vi "Configure Surge-Drop Duration.vi"(0 "VISA resource name":refnum<visa-resource-name>, 5 "Surge Drop Duration (0 ms)":dbl min=0.0 max=99.0, 11 "error in (no error)":errorcluster) -> (4 "VISA resource name out":refnum<visa-resource-name>, 15 "error out":errorcluster)   [LabVIEW 2020, in "eec 6700.lvlib"]
doc: "Sets <B>surge drop duration</B> of the power source instrument.\n\n<B>Range</B> : \nIf Surge Drop Continuous = ON : 0 ~ 20ms\nIf Surge Drop Continuous = OFF : 0 ~ 99ms\n\nThe Surge Drop-Time parameter setting configures the overall time duration of the surge or drop voltage. For example if the Surge Drop-Site is 50 milliseconds; the output voltage is 120 volts; the surge voltage is 150 volts; and the Surge Drop-Time is 20 milliseconds when the sine wave reaches the 50 millisecond point (180º) the voltage will surge to 150 volts. This surge will hold for 20 milliseconds before the voltage output returns to 120 volts"
uses:
  <instrlib>/eec 6700/eec 6700.lvlib
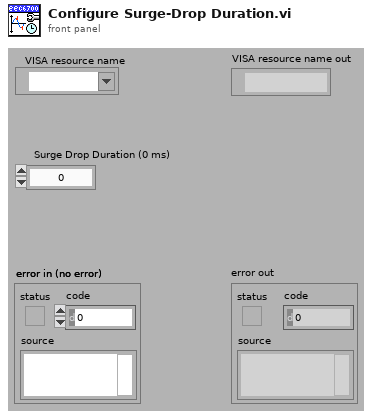
[diagram p1: front panel]
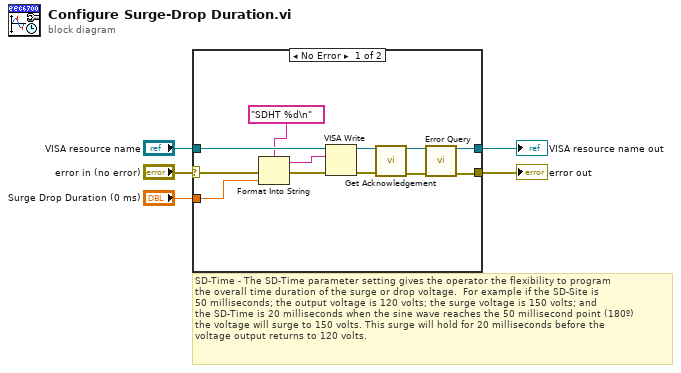
[diagram p0: block diagram]
diagram:
  # "SD-Time - The SD-Time parameter setting gives the operator the flexibility to program \nthe overall time duration of the surge or drop voltage.  For example if the SD-Site is \n50 milliseconds; the output voltage is 120 volts; the surge voltage is 150 volts; and \nthe SD-Time is 20 milliseconds when the sine wave reaches the 50 millisecond point (180º) \nthe voltage will surge to 150 volts. This surge will hold for 20 milliseconds before the \nvoltage output returns to 120 volts."
  n1 = case shown="No Error" "error in (no error)" {
    selector: "error in (no error)" -> [w11 w19]
    tunnel: [w12 w19] -> w5
    tunnel: [w13 w18] -> w4
    tunnel: "VISA resource name" -> [w17 w18]
    tunnel: "Surge Drop Duration (0 ms)" -> [w16 _]
    frame No Error {
      n2 = Format Into String(format string="SDHT %d\n" ("Command"), error in=w11, w16) -> (resulting string=w15:string, error out=w10:errorcluster)  [unwired: 1 in]
      n3 = VISA Write(VISA resource name=w17, write buffer=w15, error in (no error)=w10) -> (VISA resource name out=w7:refnum<visa-resource-name>, error out=w6:errorcluster)  [unwired: 1 out]
      n4 = call <instrlib>:"Get Acknowledgement.vi"("VISA resource name"=w7, "error in (no error)"=w6) -> ("VISA resource name out"=w8:refnum<visa-resource-name>, "error out"=w9:errorcluster)  [unwired: 12 in]
      n5 = call <instrlib>:"Error Query.vi"("VISA resource name"=w8, "error in (no error)"=w9) -> ("VISA resource name out"=w13:refnum<visa-resource-name>, "error out"=w12:errorcluster)  [unwired: 10 in, 2 out]
    }
    frame Error {
    }
  }
  "error out" <- w5
  "VISA resource name out" <- w4
